vi "WPI_CompressorOpen.vi"(0 "Pressure Switch Digital Module (Module 1)":T4, 5 "Pressure Switch DIO Channel":T3, 7 "Relay Digital Module (Module 1)":T4, 9 "Relay Channel":T6, 11 "error in (no error)":errorcluster) -> (4 "CompressorDevRef":T1={"DevStatus"={"status"=FALSE, "code"=0, "source"=""}, "DigitalInputDevRef"={"DevStatus"={"status"=FALSE, "code"=0, "source"=""}, "DIO Channel"=enum."DIO 1", "Digital Module"=enum."Digital Module 1"}, "RelayDevRef"={"DevStatus"={"status"=FALSE, "code"=0, "source"=""}, "Relay Channel"=enum."Invalid", "Digital Module"=enum."Digital Module 1", "Relay Direction"=enum."Both directions"}}, 15 "error out":errorcluster)   [LabVIEW 2014]
doc: "Opens a reference to the compressor you define. You must open a reference before using any other VIs on this palette. After you open a reference to the compressor, you can use the Start and Stop VIs to enable and disable the compressor monitoring and control. You also need to place a Run VI into periodic tasks and pass it the compressor reference.\n\nThis software is licensed. Open the labview\\readme\\WPI Robotics Library Open Source License.txt file for more information."
uses:
  <vilib>/Rock Robotics/SystemInterfaces/DIO/FPGA_DIOChannel.ctl
  <vilib>/Rock Robotics/SystemInterfaces/DIO/FPGA_DIORelayChannel.ctl
  <vilib>/Rock Robotics/SystemInterfaces/Typedef/FPGA_TypedefDigitalModule.ctl
  <vilib>/Rock Robotics/WPI/Compressor/WPI_CompressorDevRef.ctl
  <vilib>/Rock Robotics/WPI/DigitalInput/WPI_DigitalInputDevRef.ctl
  <vilib>/Rock Robotics/WPI/Relay/WPI_RelayDevRef.ctl
  <vilib>/Rock Robotics/WPI/Relay/WPI_RelayDirection.ctl
  <vilib>/Rock Robotics/SystemInterfaces/NetworkCommunication/NetComm_UsageReport_ResourceType.ctl
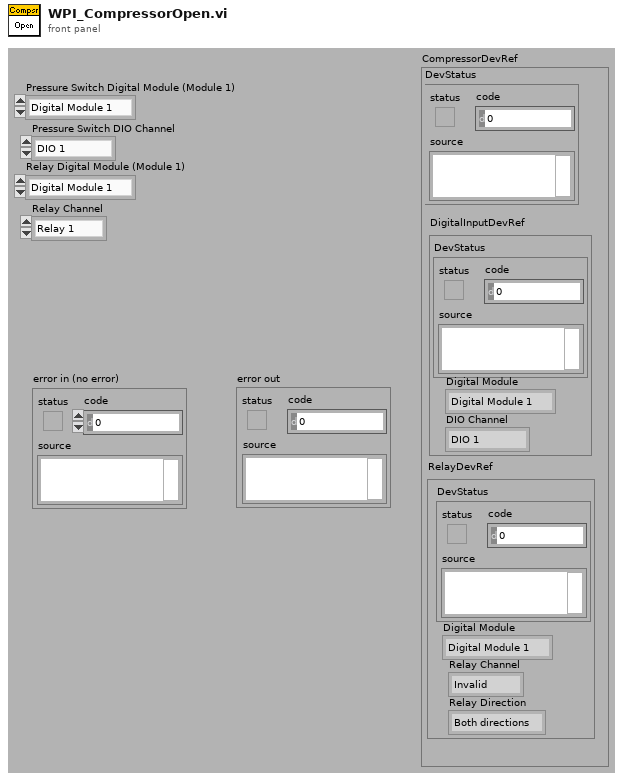
[diagram p1: front panel]
types:
  T1 = typedef "WPI_CompressorDevRef.ctl" = cluster{"DevStatus":errorcluster, "DigitalInputDevRef":T2, "RelayDevRef":T5}
  T2 = typedef "WPI_DigitalInputDevRef.ctl" = cluster{"DevStatus":errorcluster, "DIO Channel":T3, "Digital Module":T4}
  T3 = typedef "FPGA_DIOChannel.ctl" = enum8{"DIO 1", "DIO 2", "DIO 3", "DIO 4", "DIO 5", "DIO 6", "DIO 7", "DIO 8", "DIO 9", "DIO 10", "DIO 11", "DIO 12", "DIO 13", "DIO 14", "Invalid"}
  T4 = typedef "FPGA_TypedefDigitalModule.ctl" = enum16{"Digital Module 1", "Digital Module 2"}
  T5 = typedef "WPI_RelayDevRef.ctl" = cluster{"DevStatus":errorcluster, "Relay Channel":T6, "Digital Module":T4, "Relay Direction":T7}
  T6 = typedef "FPGA_DIORelayChannel.ctl" = enum8{"Relay 1", "Relay 2", "Relay 3", "Relay 4", "Relay 5", "Relay 6", "Relay 7", "Relay 8", "Invalid"}
  T7 = typedef "WPI_RelayDirection.ctl" = enum16{"Both directions", "Forward only", "Reverse only"}
  T8 = typedef "NetComm_UsageReport_ResourceType.ctl" = enum8{"Controller", "Module", "Language", "CANPlugin", "Accelerometer", "ADXL345", "AnalogChannel", "AnalogTrigger", "AnalogTriggerOutput", "CANJaguar", "Compressor", "Counter", "Dashboard", "DigitalInput", "DigitalOutput", "DriverStationCIO", "DriverStationEIO", "DriverStationLCD", "Encoder", "GearTooth", "Gyro", "I2C", "Framework", "Jaguar", "Joystick", "Kinect", "KinectStick", "PIDController", "Preferences", "PWM", "Relay", "RobotDrive", "SerialPort", "Servo", "Solenoid", "SPI", "Task", "Ultrasonic", "Victor", "Button", "Command", "AxisCamera", "PCVideoServer", "SmartDashboard", "Talon", "HiTechnicColorSensor", "HiTechnicAccel", "HiTechnicCompass", "SRF08"}
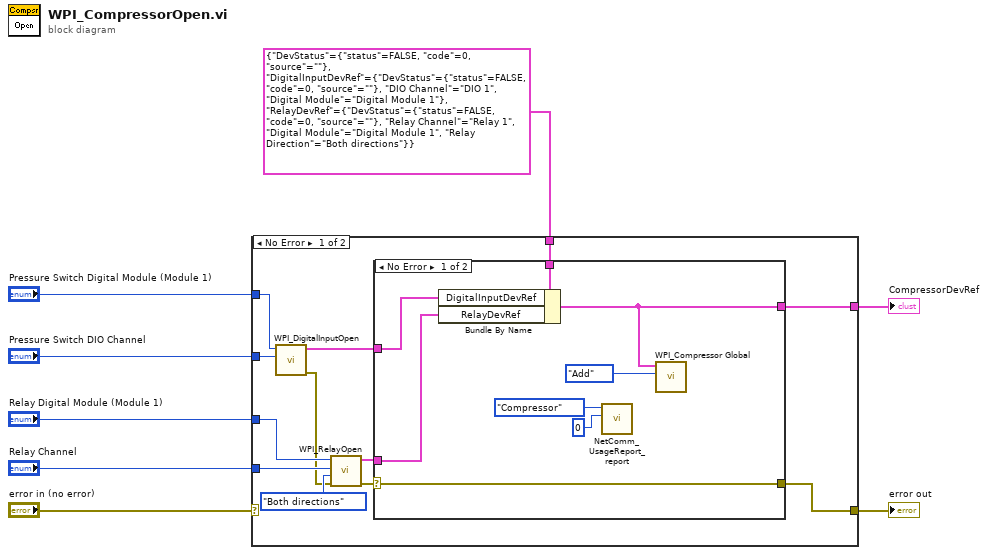
[diagram p0: block diagram]
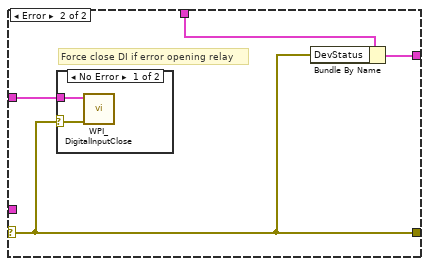
[diagram p2: hidden frame]
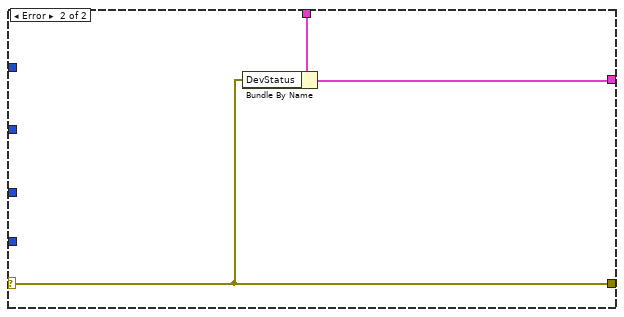
[diagram p4: hidden frame]
diagram:
  n1 = case shown="No Error" "error in (no error)" {
    selector: "error in (no error)" -> [_ w35]
    tunnel: "Pressure Switch DIO Channel" -> [w20 _]
    tunnel: "Relay Channel" -> [w19 _]
    tunnel: [w13 w35] -> w6
    tunnel: "Pressure Switch Digital Module (Module 1)" -> [w18 _]
    tunnel: "Relay Digital Module (Module 1)" -> [w17 _]
    tunnel: T1 {"DevStatus"={"status"=FALSE, "code"=0, "source"=""}, "DigitalInputDevRef"={"DevStatus"={"status"=FALSE, "code"=0, "source"=""}, "DIO Channel"=enum."DIO 1", "Digital Module"=enum."Digital Module 1"}, "RelayDevRef"={"DevStatus"={"status"=FALSE, "code"=0, "source"=""}, "Relay Channel"=enum."Relay 1", "Digital Module"=enum."Digital Module 1", "Relay Direction"=enum."Both directions"}} ("CompressorDevRef") -> [w14 w37]
    tunnel: [w9 w36] -> w1
    frame No Error {
      n2 = call <vilib>:"WPI_DigitalInputOpen.vi"("DIO Channel"=w20, "Digital Module (Module 1)"=w18) -> ("error out"=w10:errorcluster, "DigitalInputDevRef"=w16:T2)  [unwired: 1 in, 7 out]
      n3 = call <vilib>:"WPI_RelayOpen.vi"("error in (no error)"=w10, "Relay Direction"=WPI_RelayDirection."Both directions" ("RelayDirection"), "Relay Channel"=w19, "Digital Module (Module 1)"=w17) -> ("error out"=w11:errorcluster, "RelayDevRef"=w15:T5)  [unwired: 6 out]
      n4 = case shown="No Error" w11 {
        selector: w11 -> [w25 w30]
        tunnel: w16 -> [w26 w32]
        tunnel: w15 -> [w27 _]
        tunnel: [w25 w30] -> w13
        tunnel: w14 -> [w28 w31]
        tunnel: [w23 w29] -> w9
        frame No Error {
          n5 = Bundle By Name(cluster=w28, "DigitalInputDevRef"=w26, "RelayDevRef"=w27) -> (w23:T1)
          n6 = call <vilib>:"NetComm_UsageReport_report.vi"("Instance Number"=u8 0, "Resource Type"=NetComm_UsageReport_ResourceType."Compressor") -> ()  [unwired: 10 in]
          n7 = call <vilib>:"WPI_Compressor Global.vi"("Operation"=enum16{"Read", "Write", "Add", "Remove"}."Add", "CompressorDevRef"=w23) -> ()  [unwired: 8 in, 2 out]
        }
        frame Error {
          # "Force close DI if error opening relay"
          n8 = case shown="No Error" w30 {
            selector: w30 -> [w33 _]
            tunnel: w32 -> [w34 _]
            frame No Error {
              n9 = call <vilib>:"WPI_DigitalInputClose.vi"("error in (no error)"=w33, "DigitalInputDevRef"=w34) -> ()  [unwired: 10 out]
            }
            frame Error {
            }
          }
          n10 = Bundle By Name(cluster=w31, "DevStatus"=w30) -> (w29:T1)
        }
      }
    }
    frame Error {
      n11 = Bundle By Name(cluster=w37, "DevStatus"=w35) -> (w36:T1)
    }
  }
  "error out" <- w6
  "CompressorDevRef" <- w1
